vi "Write TDMS File.vi"   [LabVIEW 2020]
panel:
  # "This example writes a simulated signal to a TDMS file. \n\nInstructions:\n1. Run this VI\n2. Select a place to save your TDMS File\n3. Use the Read TDMS example to view the data."
types:
  T1 = enum16{"open", "open or create", "create or replace", "create", "open (read-only)"}
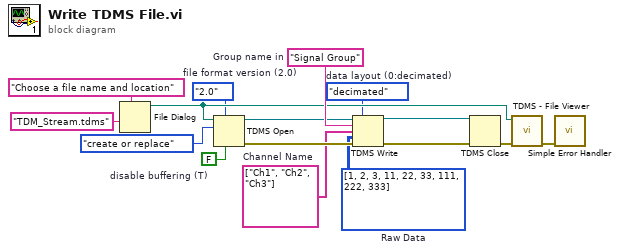
[diagram p0: block diagram]
diagram:
  w1 = enum16{"decimated", "interleaved"}."decimated"  # data layout (0:decimated)
  w2 = string[] ["Ch1", "Ch2", "Ch3"]  # Channel Name
  w3 = i32[][] [[1, 2, 3], [11, 22, 33], [111, 222, 333]]  # Raw Data
  w4 = enum16{"1.0", "2.0"}."2.0"  # file format version (2.0)
  w5 = FALSE  # disable buffering (T)
  w12 = "Signal Group"  # Group name in
  n1 = File Dialog(7:"Choose a file name and location" ("prompt"), 9:"TDM_Stream.tdms" ("default name")) -> (3:w6:path)  [unwired: 1 in, 7 out]
  n2 = TDMS Open(6:w5, 7:w4, 10:T1."create or replace" ("operation"), 11:w6) -> (0:w7:errorcluster, 3:w8:refnum<k34>)  [unwired: 3 in]
  n3 = TDMS Write(0:w8, 1:w1, 5:w12, 7:w2, 9:w3, 11:w7) -> (4:w16:refnum<k34>, 15:w13:errorcluster)  [unwired: 2 out]
  n4 = TDMS Close(8:w13, 11:w16) -> (0:w15:errorcluster)  [unwired: 1 out]
  n5 = call <vilib>:"TDMS - File Viewer.vi"("error in (no error)"=w15, "file path"=w6) -> ("error out"=w14:errorcluster)  [unwired: 5 out]
  n6 = call <vilib>:"Simple Error Handler.vi"("error in (no error)"=w14) -> ()  [unwired: 1 in, 8 out]
